vi "Is Test Case Predicate benchmark.vi"() -> ()   [LabVIEW 2020]
uses:
  <vilib>/Astemes/LUnit/Test Case.lvclass
panel:
  out "x-y":u32
  out "Array":path[](array[path])
  in  "LabVIEW Class Path":path
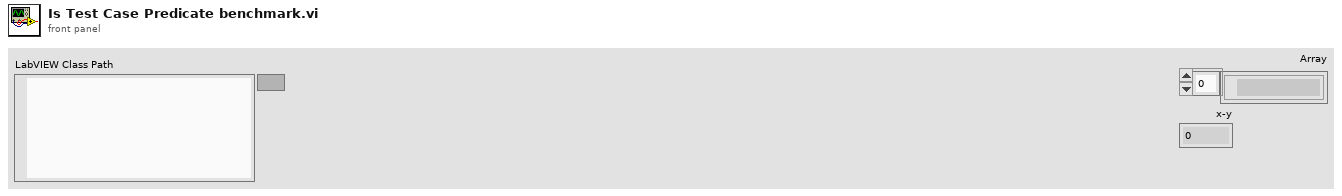
[diagram p1: front panel]
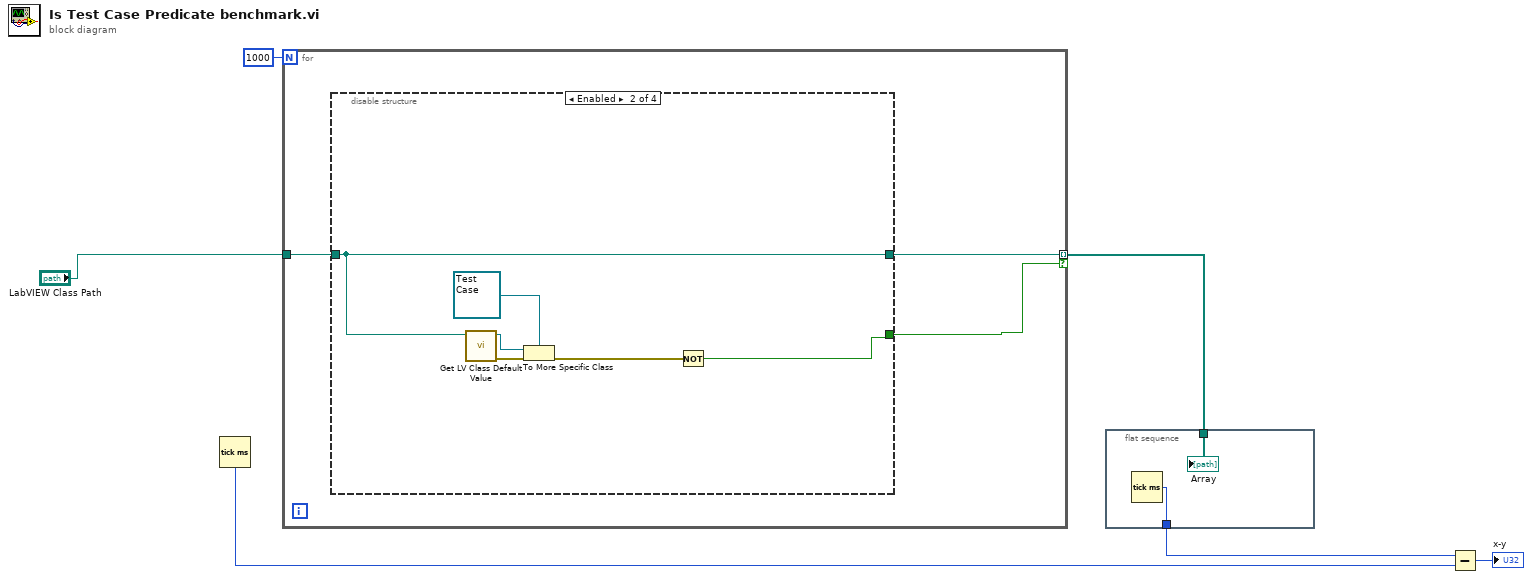
[diagram p0: block diagram]
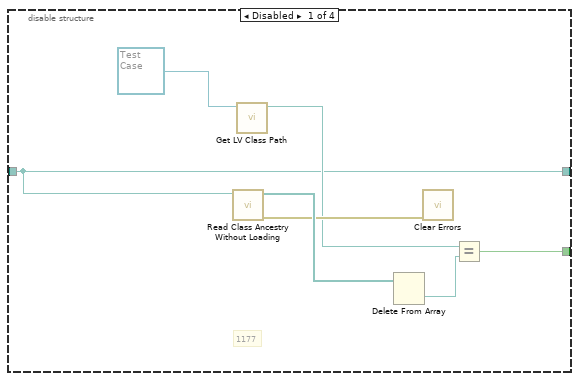
[diagram p2: hidden frame]
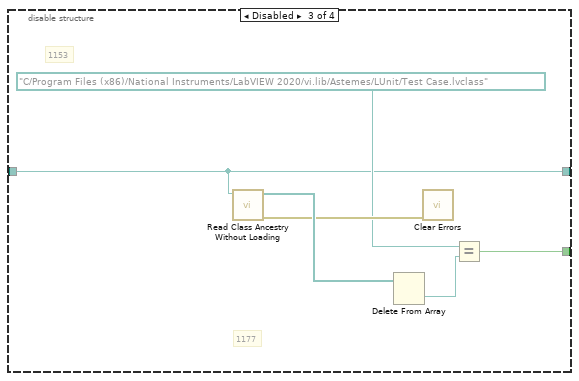
[diagram p3: hidden frame]
diagram:
  n1 = Tick Count (ms)() -> (millisecond timer value=w4:u32)
  n2 = for {
    N: 1000 -> [_]
    tunnel: [w9] -> w3 mode=indexing if=w8
    tunnel: "LabVIEW Class Path" -> [w7]
    n3 = disable-structure shown="Enabled" {
      disable-tunnel: [w10 w22 w23 _] -> w9
      disable-tunnel: [w12 w17 w25 _] -> w8
      disable-tunnel: w7 -> [w10 w22 w23 _]
      frame Disabled {
        # "1177"
        n4 = call <vilib>:"Read Class Ancestry Without Loading.vi"("LabVIEW Class Path"=w10) -> ("error out"=w14:errorcluster, "Class Ancestry"=w15:path[])  [unwired: 9 in]
        n5 = call <vilib>:"Get LV Class Path.vi"("object"=refnum<class "Test Case.lvclass"> refnum ("Test Case.lvclass")) -> ("class path"=w13:path)  [unwired: 9 in, 1 out]
        n6 = Delete From Array(array=w15) -> (deleted portion=w16:path)  [unwired: 2 in, 1 out]
        n7 = call <vilib>:"Clear Errors.vi"("error in (no error)"=w14) -> ()  [unwired: 5 in, 2 out]
        n8 = Equal?(x=w13, y=w16) -> (x = y?=w12:bool)
      }
      frame Enabled {
        n9 = call <vilib>:"Get LV Class Default Value.vi"("class path"=w22) -> ("error out"=w21:errorcluster, "object"=w20:refnum<class>)  [unwired: 9 in]
        n10 = To More Specific Class(target class=refnum<class "Test Case.lvclass"> refnum ("Test Case.lvclass"), reference=w20, error in=w21) -> (error out=w18:errorcluster)  [unwired: 1 out]
        n11 = Not(x=w18) -> (.not. x?=w17:bool)
      }
      frame Disabled {
        # "1153"
        # "1177"
        n12 = call <vilib>:"Read Class Ancestry Without Loading.vi"("LabVIEW Class Path"=w23) -> ("error out"=w26:errorcluster, "Class Ancestry"=w27:path[])  [unwired: 9 in]
        n13 = Delete From Array(array=w27) -> (deleted portion=w28:path)  [unwired: 2 in, 1 out]
        n14 = call <vilib>:"Clear Errors.vi"("error in (no error)"=w26) -> ()  [unwired: 5 in, 2 out]
        n15 = Equal?(x=path "C:/Program Files (x86)/National Instruments/LabVIEW 2020/vi.lib/Astemes/LUnit/Test Case.lvclass", y=w28) -> (x = y?=w25:bool)
      }
      frame Disabled {
      }
    }
  }
  n16 = flat-sequence {
    tunnel: [w30] -> w5
    tunnel: w3 -> [w29]
    frame #0 {
      n17 = Tick Count (ms)() -> (millisecond timer value=w30:u32)
      "Array" <- w29
    }
  }
  n18 = Subtract(x=w5, y=w4) -> (x-y=→"x-y":u32)
